vi "CAD@PartTransparent__Parameter.vi"(1 "ParamterIn":string) -> (0 "ParamterOut":string)   [LabVIEW 2020]
panel:
  in  "Slide":u32(slide) scale=0.0..100.0
  in  "PartName":string(combo)
  in  "Confirm":bool
  # "CAD@PartTransparent $Part,$ColorString"
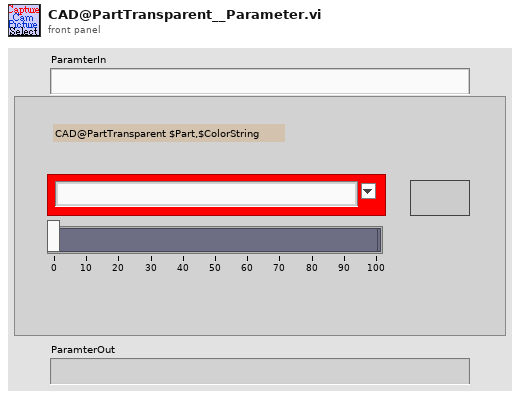
[diagram p1: front panel]
types:
  T1 = enum16{"Init", "Load Tool", "Load Part", "Get Tool Property", "Get Part Property", "Set Tool to End Matrix", "Set Part to Tool Matrix", "Calculate Part to Tool & End Matrix", "Create Part From Copy", "Delete Part"}
  T2 = cluster{"Tool Name":string[], "Part Name":string[]}
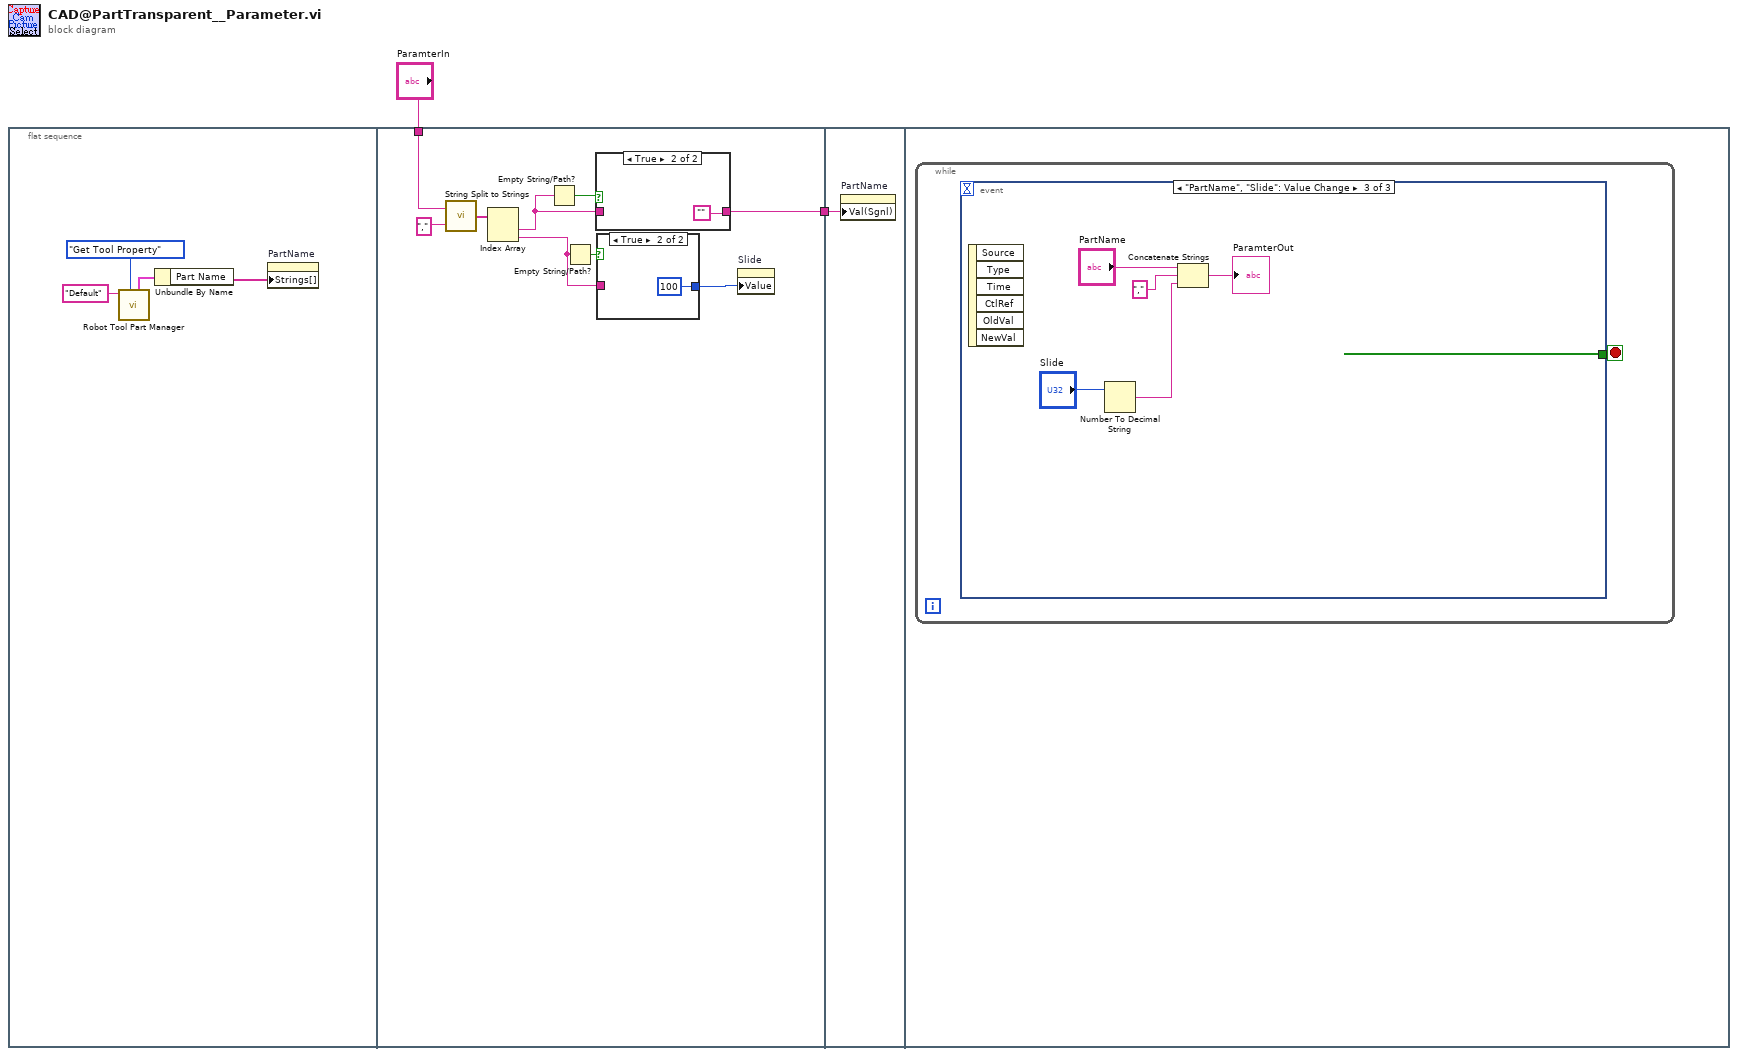
[diagram p0: block diagram]
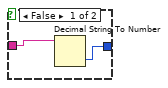
[diagram p2: hidden frame]
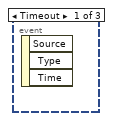
[diagram p4: hidden frame]
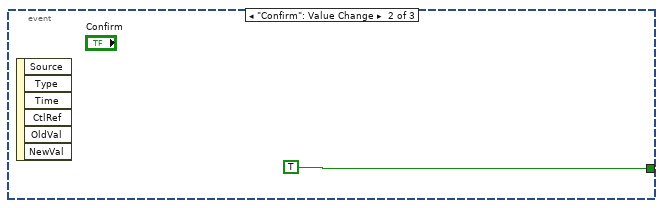
[diagram p5: hidden frame]
diagram:
  n1 = flat-sequence {
    tunnel: "ParamterIn" -> [w13]
    tunnel: [w8] -> w1
    tunnel: w1 -> [w21]
    frame #0 {
      n2 = call "Robot Tool Part Manager.vi"("CMD"=T1."Get Tool Property", "Tool / Part Name"="Default") -> ("NameList"=w4:T2)  [unwired: 4 in, 5 out]
      n3 = Unbundle By Name(w4) -> ("Part Name"=w3:string[])
      n4 = property on="PartName" class="CmbBox"("Strings[]"=w3) -> ()  [unwired: 2 in, 2 out]
    }
    frame #1 {
      n5 = call "String Split to Strings.vi"("search string/char (-)"=",", "String"=w13) -> ("Array"=w15:string[])
      n6 = Index Array(array=w15) -> (element #1=w9:string, element #2=w10:string)  [unwired: 2 in]
      n7 = Empty String/Path?(string/path=w9) -> (empty?=w12:bool)
      n8 = Empty String/Path?(string/path=w10) -> (empty?=w11:bool)
      n9 = case shown="True" w12 {
        tunnel: w9 -> [w19 _]
        tunnel: [w19 ""] -> w8
        frame False {
        }
        frame True {
        }
      }
      n10 = case shown="True" w11 {
        tunnel: w10 -> [w17 _]
        tunnel: [w16 100] -> w7
        frame False {
          n11 = Decimal String To Number(string=w17) -> (number=w16:i32)  [unwired: 2 in, 1 out]
        }
        frame True {
        }
      }
      n12 = property on="Slide" class="Slide (strict)"("Value"=w7) -> ()  [unwired: 2 in, 2 out]
    }
    frame #2 {
      n13 = property on="PartName" class="CmbBox"("Val(Sgnl)"=w21) -> ()  [unwired: 2 in, 2 out]
    }
    frame #3 {
      n14 = while {
        stop <- w22 stop-if-true
        n15 = event shown="[2] \"PartName\", \"Slide\": Value Change" {
          selector: _ -> [_ _ _]
          dyn-events: _ -> [_ _ _]
          timeout: _ -> [_ _ _]
          tunnel: [_ TRUE _] -> w22
          event Timeout {
            n16 = event-data() -> ()  [unwired: 1 in, 3 out]
          }
          event "Confirm": Value Change {
            n17 = event-data() -> ()  [unwired: 1 in, 6 out]
          }
          event "PartName", "Slide": Value Change {
            n18 = event-data() -> ()  [unwired: 1 in, 6 out]
            n19 = Number To Decimal String(number="Slide") -> (decimal integer string=w24:string)  [unwired: 1 in]
            n20 = Concatenate Strings("PartName", "," ("element"), w24) -> (→"ParamterOut":string)
          }
        }
      }
    }
  }
